vi "Move Element.vi"(8 "error in (no error)":errorcluster, 9 "From":i32=-1, 10 "To":i32=-1, 11 "ControlArray in":refnum<class "ControlArray.lvclass">) -> (0 "error out":errorcluster, 3 "ControlArray out":refnum<class "ControlArray.lvclass">)   [LabVIEW 2020, in "Control Array.lvlib" / "ControlArray.lvclass"]
doc: "Operates as if Delete From Array is called with the <b>From</b> index and then Insert into Array is called with the <b>To</b> index.\n\nIf an invalid <b>From</b> or <b>To</b> is specified then no move is performed."
uses:
  ControlArray.lvclass
  ControlArray.lvclass/ControlArray.ctl
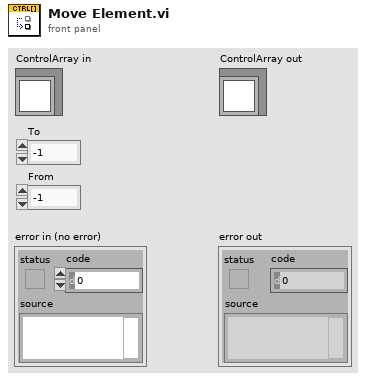
[diagram p1: front panel]
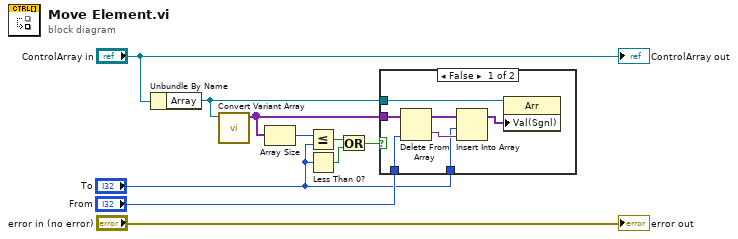
[diagram p0: block diagram]
diagram:
  n1 = Unbundle By Name("ControlArray in") -> ("Array"=w3:refnum<vi>)
  n2 = call "Convert Variant Array.vi"("Array"=w3) -> ("Variant Array"=w4:variant[])  [unwired: 9 in, 1 out]
  n3 = Array Size(array=w4) -> (size(s)=w8:i32)
  n4 = Less Or Equal?(x=w8, y="To") -> (x <= y?=w7:bool)
  n5 = Less Than 0?(x="To") -> (x < 0?=w6:bool)
  n6 = Or(x=w7, y=w6) -> (x .or. y?=w5:bool)
  n7 = case shown="False" w5 {
    tunnel: w4 -> [w14 _]
    tunnel: w3 -> [w17 _]
    tunnel: "To" -> [w12 _]
    tunnel: "From" -> [w11 _]
    frame False {
      n8 = Delete From Array(array=w14, index=w11) -> (deleted portion=w15:variant, array with subset deleted=w16:variant[])  [unwired: 1 in]
      n9 = Insert Into Array(array=w16, index=w12, new element=w15) -> (w13:variant[])
      n10 = property class="Arr"(reference=w17, "Val(Sgnl)"=w13) -> ()  [unwired: 1 in, 2 out]
    }
    frame True {
    }
  }
  "error out" <- "error in (no error)"
  "ControlArray out" <- "ControlArray in"
